vi "NoBrokenWire.vi"() -> ()   [LabVIEW 2013]
panel:
  out "Waveform Graph":dbl[](graph)
  in  "String":string
  in  "Boolean":bool
  out "Gauge":dbl(knob) scale=0.0..10.0
  out "Vertical Pointer Slide":dbl(slide) scale=0.0..100.0
  in  "Knob":dbl(knob) scale=0.0..100.0
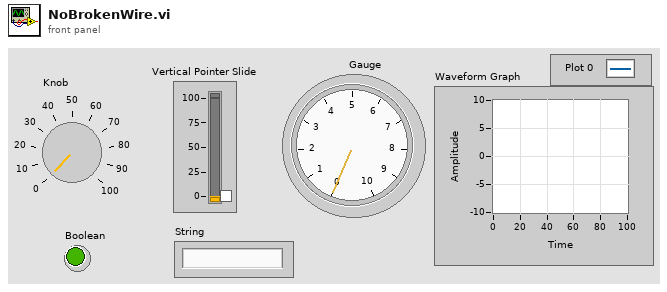
[diagram p1: front panel]
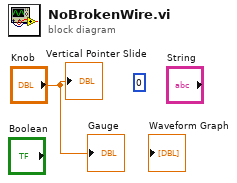
[diagram p0: block diagram]
diagram:
  (unwired) 0
  "Vertical Pointer Slide" <- "Knob"
  "Gauge" <- "Knob"
